vi "mod_AM DSB CE Demodulation (block processing).vi"(0 "x":cdb[](array[numeric]) format="%.2f", 5 "modulation index":dbl=1.0 format="%.2f", 11 "error in (no error)":errorcluster, 13 "suppress carrier ?":bool=TRUE) -> (4 "AM demod":dbl[](array[numeric]) format="%.2f", 6 "carrier amplitude":dbl format="%.2f", 15 "error out":errorcluster)   [LabVIEW 2020, in "niAMT.lvlib"]
doc: "This VI performs analog demodulation on double side band AM signal with carrier. The input signal is frequency shifted base band I-Q signal."
uses:
  <vilib>/addons/Modulation/niAMT.lvlib
  <vilib>/Analysis/baseanly.llb/Mean (DBL).vi
  <vilib>/Analysis/0measdsp.llb/Scaled Time Domain Window (DBL).vi
  <vilib>/Analysis/NI_AALBase.lvlib
  <vilib>/Analysis/NI_AALPro.lvlib
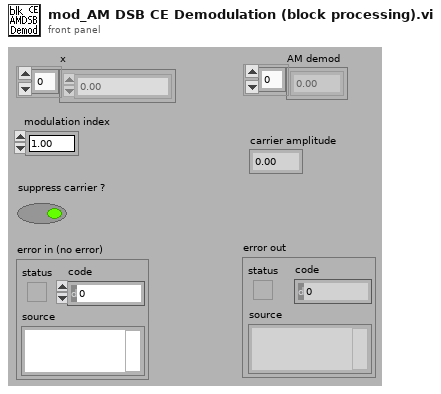
[diagram p1: front panel]
types:
  T1 = enum16{"None ", "Hanning", "Hamming", "Blackman-Harris", "Exact Blackman", "Blackman", "Flat Top", "4 Term B-Harris ", "7 Term B-Harris", "Low Sidelobe"}
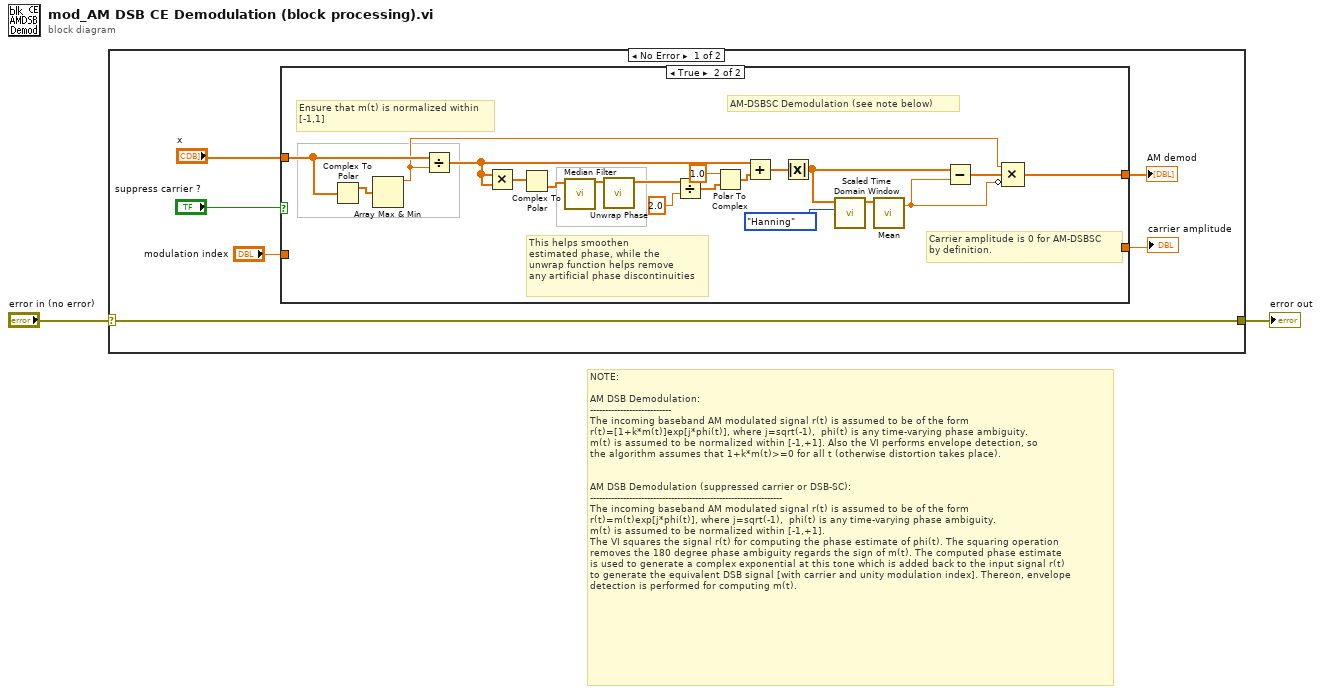
[diagram p0: block diagram]
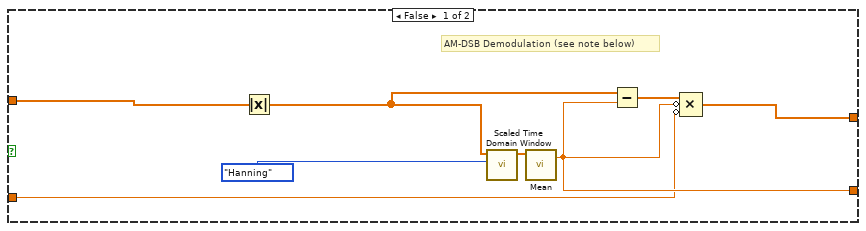
[diagram p2: hidden frame]
diagram:
  # "NOTE:\n\nAM DSB Demodulation:\n---------------------------\nThe incoming baseband AM modulated signal r(t) is assumed to be of the form\nr(t)=[1+k*m(t)]exp[j*phi(t)], where j=sqrt(-1),  phi(t) is any time-varying phase ambiguity.\nm(t) is assumed to be normalized within [-1,+1]. Also the VI performs envelope detection, so\nthe algorithm assumes that 1+k*m(t)>=0 for all t (otherwise distortion takes place).  \n\n\nAM DSB Demodulation (suppressed carrier or DSB-SC): \n----------------------------------------------------------------\nThe incoming baseband AM modulated signal r(t) is assumed to be of the form\nr(t)=m(t)exp[j*phi(t)], where j=sqrt(-1),  phi(t) is any time-varying phase ambiguity.\nm(t) is assumed to be normalized within [-1,+1].\nThe VI squares the signal r(t) for computing the phase estimate of phi(t). The squaring operation \nremoves the 180 degree phase ambiguity regards the sign of m(t). The computed phase estimate \nis used to generate a complex exponential at this tone which is added back to the input signal r(t) \nto generate the equivalent DSB signal [with carrier and unity modulation index]. Thereon, envelope \ndetection is performed for computing m(t)."
  n1 = case shown="No Error" "error in (no error)" {
    selector: "error in (no error)" -> [w3 w36]
    tunnel: [w3 w36] -> w1
    frame No Error {
      n2 = case shown="True" "suppress carrier ?" {
        tunnel: "x" -> [w16 w22]
        tunnel: [w14 w31] -> w8
        tunnel: [w11 _] -> w7
        tunnel: "modulation index" -> [w9 _]
        frame False {
          # "AM-DSB Demodulation (see note below)"
          n3 = Absolute Value(x=w16) -> (abs(x)=w12:dbl[])
          n4 = call-poly <vilib>:"Scaled Time Domain Window.vi"("window"=T1."Hanning" ("weighting window"), "X"=w12) -> ("Windowed X"=w10:dbl[])  [unwired: 1 in, 8 out]
          n5 = call-poly <vilib>:"Mean.vi"("X"=w10) -> ("mean"=w11:dbl)  [unwired: 1 out]
          n6 = Subtract(x=w12, y=w11) -> (x-y=w15:dbl[])
          n7 = Compound Arithmetic op=MULTIPLY(w15, invert w11, invert w9) -> (w14:dbl[])
        }
        frame True {
          # "Carrier amplitude is 0 for AM-DSBSC\nby definition."
          # "This helps smoothen\nestimated phase, while the\nunwrap function helps remove\nany artificial phase discontinuities"
          # "Ensure that m(t) is normalized within\n[-1,1]"
          # "AM-DSBSC Demodulation (see note below)"
          n8 = Complex To Polar(r * e^(i*theta)=w22) -> (r=w23:dbl[])  [unwired: 1 out]
          n9 = Array Max & Min(array=w23) -> (max value=w20:dbl)  [unwired: 3 out]
          n10 = Divide(x=w22, y=w20) -> (x/y=w21:cdb[])
          n11 = Multiply(x=w21, y=w21) -> (x*y=w27:cdb[])
          n12 = Complex To Polar(r * e^(i*theta)=w27) -> (theta=w18:dbl[])  [unwired: 1 out]
          n13 = call <vilib>:"Median Filter.vi"("X"=w18) -> ("Filtered X"=w19:dbl[])  [unwired: 2 in, 8 out]
          n14 = call <vilib>:"Unwrap Phase.vi"("Phase"=w19) -> ("Unwrapped Phase"=w17:dbl[])  [unwired: 1 in, 9 out]
          n15 = Divide(x=w17, y=2.0) -> (x/y=w26:dbl[])
          n16 = Polar To Complex(1:w26, 2:1.0) -> (0:w34:cdb[])
          n17 = Add(x=w21, y=w34) -> (x+y=w29:cdb[])
          n18 = Absolute Value(x=w29) -> (abs(x)=w28:dbl[])
          n19 = call-poly <vilib>:"Scaled Time Domain Window.vi"("window"=T1."Hanning", "X"=w28) -> ("Windowed X"=w33:dbl[])  [unwired: 1 in, 8 out]
          n20 = call-poly <vilib>:"Mean.vi"("X"=w33) -> ("mean"=w24:dbl)  [unwired: 1 out]
          n21 = Subtract(x=w28, y=w24) -> (x-y=w32:dbl[])
          n22 = Compound Arithmetic op=MULTIPLY(w20, w32, invert w24) -> (w31:dbl[])
        }
      }
      "AM demod" <- w8
      "carrier amplitude" <- w7
    }
    frame Error {
    }
  }
  "error out" <- w1
